vi "(16) part 2 que.vi"() -> ()   [LabVIEW 2025]
panel:
  in  "operation (0:open) 4":T1(ring)
  in  "file path (use dialog) 4":path
  out "text 4":string
  in  "operation (0:open) 3":T1(ring)
  in  "file path (use dialog) 3":path
  out "text 3":string
  in  "operation (0:open) 2":T1(ring)
  in  "file path (use dialog) 2":path
  out "text 2":string
  out "text":string
  in  "file path (use dialog)":path
  in  "operation (0:open)":T1(ring)
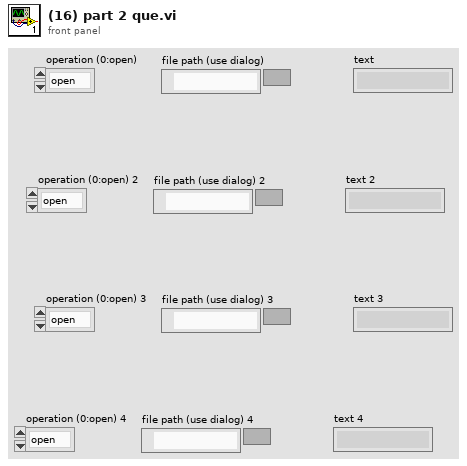
[diagram p1: front panel]
types:
  T1 = enum16{"open", "replace", "create", "open or create", "replace or create", "replace or create with confirmation"}
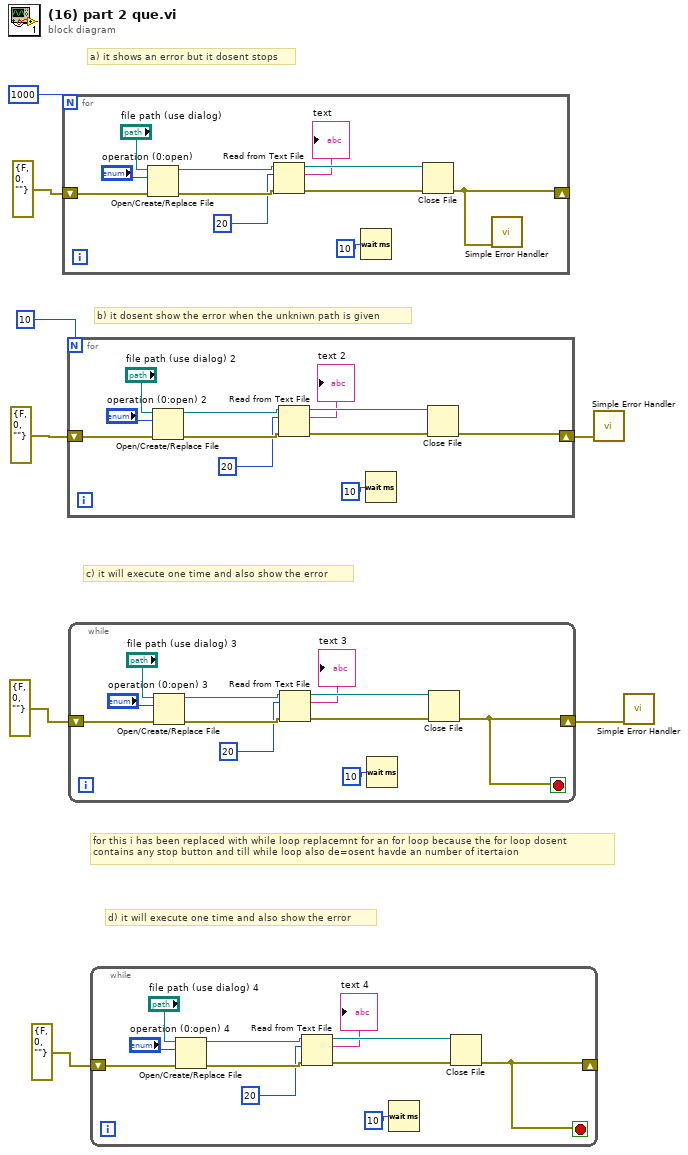
[diagram p0: block diagram]
diagram:
  # "d) it will execute one time and also show the error"
  # "for this i has been replaced with while loop replacemnt for an for loop because the for loop dosent \ncontains any stop button and till while loop also de=osent havde an number of itertaion"
  # "c) it will execute one time and also show the error"
  # "b) it dosent show the error when the unkniwn path is given"
  # "a) it shows an error but it dosent stops"
  n1 = for {
    N: 1000 -> [_]
    shift-right: [w9] -> _
    shift-left: errorcluster {"status"=FALSE, "code"=0, "source"=""} ("error constant") -> [w17]
    n2 = Open/Create/Replace File(file path (use dialog)="file path (use dialog)", error in=w17, operation (0:open)="operation (0:open)") -> (refnum out=w19:refnum<file>, error out=w16:errorcluster)  [unwired: 3 in, 1 out]
    n3 = Read from Text File(file (use dialog)=w19, count=20, error in=w16) -> (refnum out=w18:refnum<file>, text=→"text":string, error out=w15:errorcluster)  [unwired: 1 in, 1 out]
    n4 = Wait (ms)(milliseconds to wait=10) -> ()  [unwired: 1 out]
    n5 = Close File(refnum=w18, error in=w15) -> (error out=w9:errorcluster)  [unwired: 1 out]
    n6 = call <vilib>:"Simple Error Handler.vi"("error in (no error)"=w9) -> ()  [unwired: 4 in, 5 out]
  }
  n7 = for {
    N: 10 -> [_]
    shift-right: [w20] -> w4
    shift-left: errorcluster {"status"=FALSE, "code"=0, "source"=""} ("error constant") -> [w28]
    n8 = Open/Create/Replace File(file path (use dialog)="file path (use dialog) 2", error in=w28, operation (0:open)="operation (0:open) 2") -> (refnum out=w30:refnum<file>, error out=w27:errorcluster)  [unwired: 3 in, 1 out]
    n9 = Read from Text File(file (use dialog)=w30, count=20, error in=w27) -> (refnum out=w29:refnum<file>, text=→"text 2":string, error out=w26:errorcluster)  [unwired: 1 in, 1 out]
    n10 = Wait (ms)(milliseconds to wait=10) -> ()  [unwired: 1 out]
    n11 = Close File(refnum=w29, error in=w26) -> (error out=w20:errorcluster)  [unwired: 1 out]
  }
  n12 = while {
    shift-right: [w31] -> w2
    shift-left: errorcluster {"status"=FALSE, "code"=0, "source"=""} ("error constant") -> [w39]
    stop <- w31 stop-if-true
    n13 = Open/Create/Replace File(file path (use dialog)="file path (use dialog) 3", error in=w39, operation (0:open)="operation (0:open) 3") -> (refnum out=w41:refnum<file>, error out=w38:errorcluster)  [unwired: 3 in, 1 out]
    n14 = Read from Text File(file (use dialog)=w41, count=20, error in=w38) -> (refnum out=w40:refnum<file>, text=→"text 3":string, error out=w37:errorcluster)  [unwired: 1 in, 1 out]
    n15 = Wait (ms)(milliseconds to wait=10) -> ()  [unwired: 1 out]
    n16 = Close File(refnum=w40, error in=w37) -> (error out=w31:errorcluster)  [unwired: 1 out]
  }
  n17 = while {
    shift-right: [w42] -> _
    shift-left: errorcluster {"status"=FALSE, "code"=0, "source"=""} ("error constant") -> [w50]
    stop <- w42 stop-if-true
    n18 = Open/Create/Replace File(file path (use dialog)="file path (use dialog) 4", error in=w50, operation (0:open)="operation (0:open) 4") -> (refnum out=w52:refnum<file>, error out=w49:errorcluster)  [unwired: 3 in, 1 out]
    n19 = Read from Text File(file (use dialog)=w52, count=20, error in=w49) -> (refnum out=w51:refnum<file>, text=→"text 4":string, error out=w48:errorcluster)  [unwired: 1 in, 1 out]
    n20 = Wait (ms)(milliseconds to wait=10) -> ()  [unwired: 1 out]
    n21 = Close File(refnum=w51, error in=w48) -> (error out=w42:errorcluster)  [unwired: 1 out]
  }
  n22 = call <vilib>:"Simple Error Handler.vi"("error in (no error)"=w4) -> ()  [unwired: 4 in, 5 out]
  n23 = call <vilib>:"Simple Error Handler.vi"("error in (no error)"=w2) -> ()  [unwired: 4 in, 5 out]
